vi "RSZVB Set Virtual Transform Balanced State.vi"(6 "Logical Port Number (1)":i32=1, 7 "State (F: Off)":bool, 8 "error in (no error)":errorcluster {"code" format="%.0x"}, 9 "Function Type (0: Deembedding)":i32(ring) items=["Deembedding", "Embedding"], 10 "Channel (1)":i32=1, 11 "VISA session":refnum<visa-resource-name>) -> (0 "error out":errorcluster {"code" format="%.0x"}, 3 "dup VISA session":refnum<visa-resource-name>)   [LabVIEW 2011]
doc: "This VI enables or disables the deembedding/embedding VI for balanced ports.\n\nRemote-control command(s):\nCALCulate<Ch>:TRANsform:VNETworks:BALanced:DEEMbedding<Log_pt>[:STATe] <Boolean> \nCALCulate<Ch>:TRANsform:VNETworks:BALanced:EMBedding<Log_pt>[:STATe] <Boolean>"
uses:
  _utility/RSZVB Global Data.vi
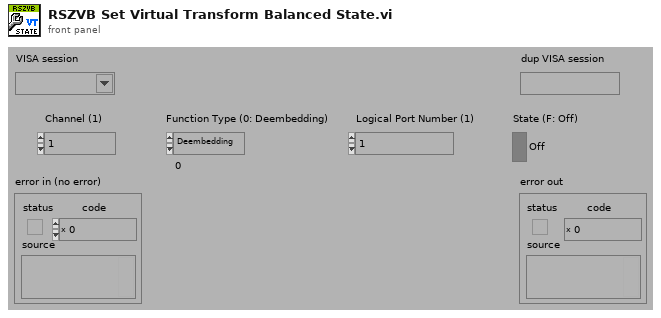
[diagram p1: front panel]
types:
  T1 = cluster{"Error Checking (T: On)":bool, "Installed Options":string[], "Data Valid?":bool, "Ports":i32, "Model":string[], "Option Checking (T: On)":bool}[]
  T2 = cluster{"Error Checking (T: On)":bool, "Installed Options":string[], "Data Valid?":bool, "Ports":i32, "Model":string[], "Option Checking (T: On)":bool}
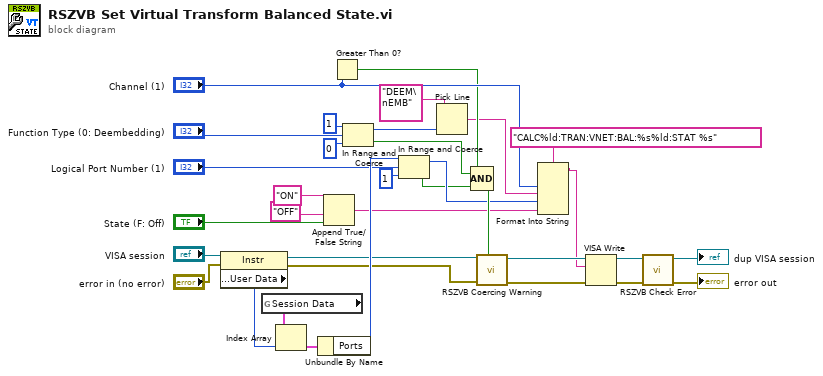
[diagram p0: block diagram]
diagram:
  n1 = property class="Instr"(reference="VISA session", error in="error in (no error)") -> (reference out=w18:refnum<visa-resource-name>, error out=w19:errorcluster, "General Settings:User Data"=w25:u32)
  n2 = global read "RSZVB Global Data.vi" "Session Data"() -> (w24:T1)
  n3 = Index Array(array=w24, index=w25) -> (element=w23:T2)
  n4 = Unbundle By Name(w23) -> ("Ports"=w22:i32)
  n5 = Append True/False String(1:"State (F: Off)", 2:"OFF", 3:"ON") -> (0:w5:string)  [unwired: 1 in]
  n6 = Greater Than 0?(x="Channel (1)") -> (x > 0?=w13:bool)
  n7 = In Range and Coerce(upper limit=1 ("lower limit"), x="Function Type (0: Deembedding)", lower limit=0) -> (coerced(x)=w3:i32, In Range?=w10:bool)
  n8 = In Range and Coerce(upper limit=w22, x="Logical Port Number (1)", lower limit=1) -> (coerced(x)=w9:i32, In Range?=w1:bool)
  n9 = Pick Line(multi-line string="DEEM\nEMB", line index=w3) -> (output string=w2:string)  [unwired: 1 in]
  n10 = Compound Arithmetic op=AND(w13, w10, w1) -> (w12:bool)
  n11 = call "RSZVB Coercing Warning.vi"("In Range?"=w12, "error in (no error)"=w19, "VISA session"=w18) -> ("error out"=w33:errorcluster, "dup VISA session"=w34:refnum<visa-resource-name>)  [unwired: 7 in]
  n12 = Format Into String(format string="CALC%ld:TRAN:VNET:BAL:%s%ld:STAT %s", "Channel (1)", w2, w9, w5) -> (resulting string=w29:string)  [unwired: 2 in, 1 out]
  n13 = VISA Write(VISA resource name=w34, write buffer=w29, error in (no error)=w33) -> (VISA resource name out=w31:refnum<visa-resource-name>, error out=w32:errorcluster)  [unwired: 1 out]
  n14 = call "RSZVB Check Error.vi"("error in (no error)"=w32, "VISA session"=w31) -> ("error out"=→"error out":errorcluster, "dup VISA session"=→"dup VISA session":refnum<visa-resource-name>)  [unwired: 8 in]
